vi "S4GUI_002.vi"(7 "Tab ObsEng":enum32{"Obs", "CCD modes", "Eng"}(tab)) -> ()   [LabVIEW 2018] (continued)
            n1927 = call-dynamic "Write sequencia_ant.vi"("error in (no error)"=w3775, "sequencia_ant"=w3776, "Opt_Selector in"=w3778) -> ("error out"=w3774:errorcluster, "Opt_Selector out"=w3777:refnum<class "Opt_Selector.lvclass">)  [unwired: 7 in]
            n1928 = local write "P8"(w3783) -> ()
            n1929 = local write "P9"(w3783) -> ()
            n1930 = local write "P10"(w3783) -> ()
            n1931 = local write "P11"(w3783) -> ()
            n1932 = local write "P12"(w3781) -> ()
            n1933 = local write "P13"(w3781) -> ()
            n1934 = local write "P14"(w3781) -> ()
            n1935 = local write "P15"(w3781) -> ()
          }
          frame 1 {
            w3787 = u16 255 ("sequencia")
            w3794 = FALSE ("P0")
            w3795 = TRUE ("P0")
            w3796 = FALSE ("P0")
            w3797 = TRUE ("P0")
            # "0000 0000 1111 1111 = 255"
            n1936 = local write "P0"(w3797) -> ()
            n1937 = local write "P1"(w3797) -> ()
            n1938 = local write "P2"(w3797) -> ()
            n1939 = local write "P3"(w3797) -> ()
            n1940 = local write "P4"(w3795) -> ()
            n1941 = local write "P5"(w3795) -> ()
            n1942 = local write "P6"(w3795) -> ()
            n1943 = local write "P7"(w3795) -> ()
            n1944 = call-dynamic "Write sequencia.vi"("error in (no error)"=w3792, "sequencia"=w3787, "Opt_Selector in"=w3793) -> ("error out"=w3789:errorcluster, "Opt_Selector out"=w3791:refnum<class "Opt_Selector.lvclass">)  [unwired: 7 in]
            n1945 = local write "P8"(w3796) -> ()
            n1946 = local write "P9"(w3796) -> ()
            n1947 = local write "P10"(w3796) -> ()
            n1948 = local write "P11"(w3796) -> ()
            n1949 = local write "P12"(w3794) -> ()
            n1950 = local write "P13"(w3794) -> ()
            n1951 = local write "P14"(w3794) -> ()
            n1952 = local write "P15"(w3794) -> ()
            n1953 = call-dynamic "Write sequencia_ant.vi"("error in (no error)"=w3789, "sequencia_ant"=w3787, "Opt_Selector in"=w3791) -> ("error out"=w3788:errorcluster, "Opt_Selector out"=w3790:refnum<class "Opt_Selector.lvclass">)  [unwired: 7 in]
          }
          frame 2 {
            w3800 = u16 15 ("sequencia")
            w3807 = FALSE ("P0")
            w3808 = FALSE ("P0")
            w3809 = FALSE ("P0")
            w3810 = TRUE ("P0")
            # "0000 0000 0000 1111 = 15"
            n1954 = local write "P0"(w3810) -> ()
            n1955 = local write "P1"(w3810) -> ()
            n1956 = local write "P2"(w3810) -> ()
            n1957 = local write "P3"(w3810) -> ()
            n1958 = local write "P4"(w3808) -> ()
            n1959 = local write "P5"(w3808) -> ()
            n1960 = local write "P6"(w3808) -> ()
            n1961 = local write "P7"(w3808) -> ()
            n1962 = call-dynamic "Write sequencia.vi"("error in (no error)"=w3805, "sequencia"=w3800, "Opt_Selector in"=w3806) -> ("error out"=w3802:errorcluster, "Opt_Selector out"=w3804:refnum<class "Opt_Selector.lvclass">)  [unwired: 7 in]
            n1963 = call-dynamic "Write sequencia_ant.vi"("error in (no error)"=w3802, "sequencia_ant"=w3800, "Opt_Selector in"=w3804) -> ("error out"=w3801:errorcluster, "Opt_Selector out"=w3803:refnum<class "Opt_Selector.lvclass">)  [unwired: 7 in]
            n1964 = local write "P8"(w3809) -> ()
            n1965 = local write "P9"(w3809) -> ()
            n1966 = local write "P10"(w3809) -> ()
            n1967 = local write "P11"(w3809) -> ()
            n1968 = local write "P12"(w3807) -> ()
            n1969 = local write "P13"(w3807) -> ()
            n1970 = local write "P14"(w3807) -> ()
            n1971 = local write "P15"(w3807) -> ()
          }
          frame 3 {
            w3814 = u16 3855 ("sequencia")
            w3820 = FALSE ("P0")
            w3821 = FALSE ("P0")
            w3822 = TRUE ("P0")
            w3823 = TRUE ("P0")
            # "0000 1111 0000 1111 = 3855"
            n1972 = local write "P0"(w3823) -> ()
            n1973 = local write "P1"(w3823) -> ()
            n1974 = local write "P2"(w3823) -> ()
            n1975 = local write "P3"(w3823) -> ()
            n1976 = local write "P4"(w3821) -> ()
            n1977 = local write "P5"(w3821) -> ()
            n1978 = local write "P6"(w3821) -> ()
            n1979 = local write "P7"(w3821) -> ()
            n1980 = call-dynamic "Write sequencia.vi"("error in (no error)"=w3818, "sequencia"=w3814, "Opt_Selector in"=w3819) -> ("error out"=w3816:errorcluster, "Opt_Selector out"=w3817:refnum<class "Opt_Selector.lvclass">)  [unwired: 7 in]
            n1981 = local write "P8"(w3822) -> ()
            n1982 = local write "P9"(w3822) -> ()
            n1983 = local write "P10"(w3822) -> ()
            n1984 = local write "P11"(w3822) -> ()
            n1985 = local write "P12"(w3820) -> ()
            n1986 = local write "P13"(w3820) -> ()
            n1987 = local write "P14"(w3820) -> ()
            n1988 = local write "P15"(w3820) -> ()
            n1989 = call-dynamic "Write sequencia_ant.vi"("error in (no error)"=w3816, "sequencia_ant"=w3814, "Opt_Selector in"=w3817) -> ("error out"=w3815:errorcluster, "Opt_Selector out"=w3813:refnum<class "Opt_Selector.lvclass">)  [unwired: 7 in]
          }
          frame 4 {
            w3826 = u16 0 ("sequencia")
            w3833 = FALSE ("P0")
            w3834 = FALSE ("P0")
            w3835 = FALSE ("P0")
            w3836 = FALSE ("P0")
            n1990 = local write "P0"(w3836) -> ()
            n1991 = local write "P1"(w3836) -> ()
            n1992 = local write "P2"(w3836) -> ()
            n1993 = local write "P3"(w3836) -> ()
            n1994 = local write "P4"(w3834) -> ()
            n1995 = local write "P5"(w3834) -> ()
            n1996 = local write "P6"(w3834) -> ()
            n1997 = local write "P7"(w3834) -> ()
            n1998 = call-dynamic "Write sequencia.vi"("error in (no error)"=w3831, "sequencia"=w3826, "Opt_Selector in"=w3832) -> ("error out"=w3828:errorcluster, "Opt_Selector out"=w3830:refnum<class "Opt_Selector.lvclass">)  [unwired: 7 in]
            n1999 = call-dynamic "Write sequencia_ant.vi"("error in (no error)"=w3828, "sequencia_ant"=w3826, "Opt_Selector in"=w3830) -> ("error out"=w3827:errorcluster, "Opt_Selector out"=w3829:refnum<class "Opt_Selector.lvclass">)  [unwired: 7 in]
            n2000 = local write "P8"(w3835) -> ()
            n2001 = local write "P9"(w3835) -> ()
            n2002 = local write "P10"(w3835) -> ()
            n2003 = local write "P11"(w3835) -> ()
            n2004 = local write "P12"(w3833) -> ()
            n2005 = local write "P13"(w3833) -> ()
            n2006 = local write "P14"(w3833) -> ()
            n2007 = local write "P15"(w3833) -> ()
          }
          frame 5 {
          }
        }
        n2008 = call "Write WPROT.vi"("error in (no error)"=w3733, "Opt_Selector.lvclass"=w3740, "Instrument in"=w3739) -> ("error out"=w3742:errorcluster, "Instrument out"=w3743:refnum<class "Instrument.lvclass">)  [unwired: 7 in]
        n2009 = property on="#Pol. Seq. Done" class="Slide (strict)"(error in=w3733, "Scale.Maximum"=w3734, "Scale.Minimum"=w3732) -> ()  [unwired: 1 in, 2 out]
        n2010 = call "Write Instrument.lvclass.vi"("error in (no error)"=w3742, "Instrument.lvclass"=w3743, "S4ACS_GUI in"=w3738) -> ("error out"=w3722:errorcluster, "S4ACS_GUI out"=w3723:refnum<class "S4GUI.lvclass">)  [unwired: 7 in]
        n2011 = call "Read Instrument.lvclass.vi"("error in (no error)"=w3722, "S4ACS_GUI in"=w3723) -> ("error out"=w3727:errorcluster, "Instrument.lvclass"=w3728:refnum<class "Instrument.lvclass">, "S4ACS_GUI out"=w3731:refnum<class "S4GUI.lvclass">)  [unwired: 7 in]
        n2012 = call "Read ASEL.vi"("error in (no error)"=w3727, "Instrument in"=w3728) -> ("error out"=w3717:errorcluster, "Opt_Selector.lvclass"=w3719:refnum<class "Opt_Selector.lvclass">, "Instrument out"=w3724:refnum<class "Instrument.lvclass">)  [unwired: 7 in]
        n2013 = call "Read name_pos.vi"("error in (no error)"=w3717, "Optics in"=w3719) -> ("error out"=w3716:errorcluster, "name_pos"=w3715:string, "Optics out"=w3718:refnum<class "Opt_Selector.lvclass">)  [unwired: 7 in]
        n2014 = call "Write ASEL.vi"("error in (no error)"=w3716, "Opt_Selector.lvclass"=w3718, "Instrument in"=w3724) -> ("error out"=w3725:errorcluster, "Instrument out"=w3729:refnum<class "Instrument.lvclass">)  [unwired: 7 in]
        n2015 = case shown="\"ON\"" w3715 {
          tunnel: w3725 -> [w3748 w3759]
          tunnel: [w3748 w3755] -> w3726
          tunnel: w3729 -> [w3747 w3760]
          tunnel: [w3747 w3756] -> w3730
          frame Default {
          }
          frame "ON" {
            n2016 = call "Read WPROT.vi"("error in (no error)"=w3759, "Instrument in"=w3760) -> ("error out"=w3751:errorcluster, "Opt_Selector.lvclass"=w3758:refnum<class "Opt_Selector.lvclass">, "Instrument out"=w3757:refnum<class "Instrument.lvclass">)  [unwired: 7 in]
            n2017 = call-dynamic "Read sequencia.vi"("error in (no error)"=w3751, "Opt_Selector in"=w3758) -> ("error out"=w3750:errorcluster, "sequencia"=w3754:u16, "Opt_Selector out"=w3753:refnum<class "Opt_Selector.lvclass">)  [unwired: 7 in]
            n2018 = case shown="0" w3754 {
              tunnel: w3753 -> [w3762 w3771]
              tunnel: [w3762 w3767] -> w3752
              tunnel: w3750 -> [w3761 w3770]
              tunnel: [w3761 w3765] -> w3749
              frame Default {
              }
              frame 0 {
                n2019 = call-dynamic "Write sequencia.vi"("error in (no error)"=w3770, "sequencia"=u16 1, "Opt_Selector in"=w3771) -> ("error out"=w3766:errorcluster, "Opt_Selector out"=w3768:refnum<class "Opt_Selector.lvclass">)  [unwired: 7 in]
                n2020 = local write "P0"(TRUE ("P0")) -> ()
                n2021 = call-dynamic "Write sequencia_ant.vi"("error in (no error)"=w3766, "sequencia_ant"=u16 1, "Opt_Selector in"=w3768) -> ("error out"=w3765:errorcluster, "Opt_Selector out"=w3767:refnum<class "Opt_Selector.lvclass">)  [unwired: 7 in]
              }
            }
            n2022 = call "Write WPROT.vi"("error in (no error)"=w3749, "Opt_Selector.lvclass"=w3752, "Instrument in"=w3757) -> ("error out"=w3755:errorcluster, "Instrument out"=w3756:refnum<class "Instrument.lvclass">)  [unwired: 7 in]
          }
        }
        n2023 = call "Write Instrument.lvclass.vi"("error in (no error)"=w3726, "Instrument.lvclass"=w3730, "S4ACS_GUI in"=w3731) -> ("error out"=w3721:errorcluster, "S4ACS_GUI out"=w3720:refnum<class "S4GUI.lvclass">)  [unwired: 7 in]
      }
      event "P0", "P1", "P2", "P3", "P4", "P5", "P6", "P7", "P8", "P9", "P10", "P11", "P12", "P13", "P14", "P15": Value Change {
        w3894 = u16 5 items=["All 16 positions", "First 8 positions", "First 4 positions", "0-3 + 8-11", "Clear", "Customized"] ("Select Positions")
        # "Garantir que, quando em POLARIMETRIA, pelo menos WP1 esteja selecionado."
        # "Salva tambem em \nSequencia_ant para\no caso de repeticao."
        n2024 = event-data() -> ()  [unwired: 1 in, 6 out]
        n2025 = call "Read Instrument.lvclass.vi"("error in (no error)"=w3876, "S4ACS_GUI in"=w3877) -> ("error out"=w3871:errorcluster, "Instrument.lvclass"=w3874:refnum<class "Instrument.lvclass">, "S4ACS_GUI out"=w3875:refnum<class "S4GUI.lvclass">)  [unwired: 7 in]
        n2026 = Build Array("P0", "P1", "P2", "P3", "P4", "P5", "P6", "P7", "P8", "P9", "P10", "P11", "P12", "P13", "P14", "P15") -> (w3862:bool[])
        n2027 = call "Read WPROT.vi"("error in (no error)"=w3871, "Instrument in"=w3874) -> ("error out"=w3870:errorcluster, "Opt_Selector.lvclass"=w3872:refnum<class "Opt_Selector.lvclass">, "Instrument out"=w3873:refnum<class "Instrument.lvclass">)  [unwired: 7 in]
        n2028 = local write "Select Positions"(w3894) -> ()
        n2029 = Boolean Array To Number(Boolean array=w3862) -> (number=w3878:u32)
        n2030 = To Unsigned Word Integer(number=w3878) -> (unsigned 16bit integer=w3863:u16)
        n2031 = call-dynamic "Write sequencia.vi"("error in (no error)"=w3870, "sequencia"=w3863, "Opt_Selector in"=w3872) -> ("error out"=w3865:errorcluster, "Opt_Selector out"=w3867:refnum<class "Opt_Selector.lvclass">)  [unwired: 7 in]
        n2032 = call-dynamic "Write sequencia_ant.vi"("error in (no error)"=w3865, "sequencia_ant"=w3863, "Opt_Selector in"=w3867) -> ("error out"=w3864:errorcluster, "Opt_Selector out"=w3866:refnum<class "Opt_Selector.lvclass">)  [unwired: 7 in]
        n2033 = for {
          tunnel: w3862 -> [w3923] mode=indexing
          shift-right: [w3922] -> w3860
          shift-left: 0 -> [w3920]
          # "calcula qtd de 1s"
          n2034 = Increment(x=w3920) -> (x+1=w3921:i32)
          n2035 = Select(t=w3921, s=w3923, f=w3920) -> (s? t:f=w3922:i32)
        }
        n2036 = call "Write WPROT.vi"("error in (no error)"=w3864, "Opt_Selector.lvclass"=w3866, "Instrument in"=w3873) -> ("error out"=w3869:errorcluster, "Instrument out"=w3868:refnum<class "Instrument.lvclass">)  [unwired: 7 in]
        n2037 = call "Write Instrument.lvclass.vi"("error in (no error)"=w3869, "Instrument.lvclass"=w3868, "S4ACS_GUI in"=w3875) -> ("error out"=w3843:errorcluster, "S4ACS_GUI out"=w3844:refnum<class "S4GUI.lvclass">)  [unwired: 7 in]
        n2038 = property on="#Pol. Seq. Done" class="Slide (strict)"("Scale.Maximum"=w3860, "Scale.Minimum"=0.0 ("Scale.Range:Minimum")) -> ()  [unwired: 2 in, 2 out]
        n2039 = call "Read Instrument.lvclass.vi"("error in (no error)"=w3843, "S4ACS_GUI in"=w3844) -> ("error out"=w3849:errorcluster, "Instrument.lvclass"=w3848:refnum<class "Instrument.lvclass">, "S4ACS_GUI out"=w3845:refnum<class "S4GUI.lvclass">)  [unwired: 7 in]
        n2040 = call "Read ASEL.vi"("error in (no error)"=w3849, "Instrument in"=w3848) -> ("error out"=w3855:errorcluster, "Opt_Selector.lvclass"=w3853:refnum<class "Opt_Selector.lvclass">, "Instrument out"=w3852:refnum<class "Instrument.lvclass">)  [unwired: 7 in]
        n2041 = call "Read name_pos.vi"("error in (no error)"=w3855, "Optics in"=w3853) -> ("error out"=w3856:errorcluster, "name_pos"=w3857:string, "Optics out"=w3854:refnum<class "Opt_Selector.lvclass">)  [unwired: 7 in]
        n2042 = call "Write ASEL.vi"("error in (no error)"=w3856, "Opt_Selector.lvclass"=w3854, "Instrument in"=w3852) -> ("error out"=w3851:errorcluster, "Instrument out"=w3847:refnum<class "Instrument.lvclass">)  [unwired: 7 in]
        n2043 = case shown="\"ON\"" w3857 {
          tunnel: w3851 -> [w3896 w3907]
          tunnel: [w3896 w3903] -> w3850
          tunnel: w3847 -> [w3895 w3908]
          tunnel: [w3895 w3904] -> w3846
          frame Default {
          }
          frame "ON" {
            n2044 = call "Read WPROT.vi"("error in (no error)"=w3907, "Instrument in"=w3908) -> ("error out"=w3899:errorcluster, "Opt_Selector.lvclass"=w3906:refnum<class "Opt_Selector.lvclass">, "Instrument out"=w3905:refnum<class "Instrument.lvclass">)  [unwired: 7 in]
            n2045 = call-dynamic "Read sequencia.vi"("error in (no error)"=w3899, "Opt_Selector in"=w3906) -> ("error out"=w3898:errorcluster, "sequencia"=w3902:u16, "Opt_Selector out"=w3901:refnum<class "Opt_Selector.lvclass">)  [unwired: 7 in]
            n2046 = case shown="0" w3902 {
              tunnel: w3901 -> [w3910 w3919]
              tunnel: [w3910 w3915] -> w3900
              tunnel: w3898 -> [w3909 w3918]
              tunnel: [w3909 w3913] -> w3897
              frame Default {
              }
              frame 0 {
                n2047 = call-dynamic "Write sequencia.vi"("error in (no error)"=w3918, "sequencia"=u16 1, "Opt_Selector in"=w3919) -> ("error out"=w3914:errorcluster, "Opt_Selector out"=w3916:refnum<class "Opt_Selector.lvclass">)  [unwired: 7 in]
                n2048 = local write "P0"(TRUE ("P0")) -> ()
                n2049 = call-dynamic "Write sequencia_ant.vi"("error in (no error)"=w3914, "sequencia_ant"=u16 1, "Opt_Selector in"=w3916) -> ("error out"=w3913:errorcluster, "Opt_Selector out"=w3915:refnum<class "Opt_Selector.lvclass">)  [unwired: 7 in]
              }
            }
            n2050 = call "Write WPROT.vi"("error in (no error)"=w3897, "Opt_Selector.lvclass"=w3900, "Instrument in"=w3905) -> ("error out"=w3903:errorcluster, "Instrument out"=w3904:refnum<class "Instrument.lvclass">)  [unwired: 7 in]
          }
        }
        n2051 = call "Write Instrument.lvclass.vi"("error in (no error)"=w3850, "Instrument.lvclass"=w3846, "S4ACS_GUI in"=w3845) -> ("error out"=w3841:errorcluster, "S4ACS_GUI out"=w3842:refnum<class "S4GUI.lvclass">)  [unwired: 7 in]
      }
      event "SSM": Value Change {
        # "F: fotom.\nT: polar."
        n2052 = event-data() -> ("NewVal"=w3931:u16)  [unwired: 1 in, 5 out]
        n2053 = call-dynamic "Read mode EXPOSE.vi"("error in (no error)"=w3937, "S4GUI in"=w3938) -> ("error out"=w3936:errorcluster, "mode EXPOSE"=w3932:bool, "S4GUI out"=w3933:refnum<class "S4GUI.lvclass">)  [unwired: 7 in]
        n2054 = call "Read Instrument.lvclass.vi"("error in (no error)"=w3936, "S4ACS_GUI in"=w3933) -> ("error out"=w3935:errorcluster, "Instrument.lvclass"=w3941:refnum<class "Instrument.lvclass">, "S4ACS_GUI out"=w3940:refnum<class "S4GUI.lvclass">)  [unwired: 7 in]
        n2055 = call-dynamic "Read mode.vi"("error in (no error)"=w3935, "Instrument in"=w3941) -> ("error out"=w3934:errorcluster, "mode"=w3939:bool)  [unwired: 7 in, 1 out]
        n2056 = case shown="1" w3931 {
          tunnel: [TRUE FALSE] -> w3944
          tunnel: w3934 -> [w3950 w4177]
          tunnel: w3940 -> [w3952 w4176]
          tunnel: [w3954 w4168] -> w3943
          tunnel: [w3946 w4167] -> w3942
          tunnel: w3939 -> [_ w4157]
          tunnel: w3932 -> [_ w4155]
          tunnel: ["SYNCHRONOUS" "ASYNCHRONOUS"] -> w3924
          frame 1 {
            # "Sync mode: Os canais sao configurados para Trigger externo, desde que o SyncBox esteja conectado."
            # "Sync by Cycle"
            n2057 = call-dynamic "Read Sync Box.lvclass.vi"("error in (no error)"=w3950, "SPARC4_AC in"=w3952) -> ("error out"=w3949:errorcluster, "Sync Box.lvclass"=w3953:refnum<class "Sync Box.lvclass">, "SPARC4_AC out"=w3951:refnum<class "S4GUI.lvclass">)  [unwired: 7 in]
            n2058 = call "Read connection.vi"("error in (no error)"=w3949, "Server in"=w3953) -> ("error out"=w3948:errorcluster, "connection"=w3947:bool)  [unwired: 7 in, 1 out]
            n2059 = case shown="False" w3947 {
              tunnel: [w3957 w3974] -> w3954
              tunnel: w3951 -> [w3957 w3964]
              tunnel: w3948 -> [w3956 w3963]
              tunnel: [w3956 w3958] -> w3946
              frame False {
              }
              frame True {
                n2060 = call-dynamic "Read AcquisitionC.vi"("error in (no error)"=w3963, "S4ACS_GUI in"=w3964) -> ("error out"=w3981:errorcluster, "Acquisition.lvclass"=w3980:refnum<class "Acquisition.lvclass">)  [unwired: 7 in, 1 out]
                n2061 = call-dynamic "Read AcquisitionA.vi"("error in (no error)"=w3963, "S4ACS_GUI in"=w3964) -> ("error out"=w3984:errorcluster, "Acquisition.lvclass"=w3985:refnum<class "Acquisition.lvclass">, "S4ACS_GUI out"=w3973:refnum<class "S4GUI.lvclass">)  [unwired: 7 in]
                n2062 = call "Read AcquisitionB.vi"("error in (no error)"=w3963, "S4ACS_GUI in"=w3964) -> ("error out"=w3982:errorcluster, "Acquisition.lvclass"=w3983:refnum<class "Acquisition.lvclass">)  [unwired: 7 in, 1 out]
                n2063 = call-dynamic "Read AcquisitionD.vi"("error in (no error)"=w3963, "S4ACS_GUI in"=w3964) -> ("error out"=w3978:errorcluster, "Acquisition.lvclass"=w3979:refnum<class "Acquisition.lvclass">)  [unwired: 7 in, 1 out]
                n2064 = call-dynamic "Read enabled.vi"("error in (no error)"=w3978, "Server in"=w3979) -> ("error out"=w3987:errorcluster, "enabled"=w3986:bool, "Server out"=w3988:refnum<class "Acquisition.lvclass">)  [unwired: 7 in]
                n2065 = call-dynamic "Read enabled.vi"("error in (no error)"=w3981, "Server in"=w3980) -> ("error out"=w3990:errorcluster, "enabled"=w3989:bool, "Server out"=w3991:refnum<class "Acquisition.lvclass">)  [unwired: 7 in]
                n2066 = call-dynamic "Read enabled.vi"("error in (no error)"=w3982, "Server in"=w3983) -> ("error out"=w3993:errorcluster, "enabled"=w3992:bool, "Server out"=w3994:refnum<class "Acquisition.lvclass">)  [unwired: 7 in]
                n2067 = call-dynamic "Read enabled.vi"("error in (no error)"=w3984, "Server in"=w3985) -> ("error out"=w3996:errorcluster, "enabled"=w3995:bool, "Server out"=w3997:refnum<class "Acquisition.lvclass">)  [unwired: 7 in]
                n2068 = case shown="True" w3992 {
                  tunnel: w3994 -> [w4077 w4081]
                  tunnel: w3993 -> [w4076 w4080]
                  tunnel: [w4077 w4079] -> w3970
                  tunnel: [w4076 w4078] -> w3969
                  frame False {
                  }
                  frame True {
                    # "Ext Start"
                    # "nome do arquivo .cfg"
                    # "seção no arquivo .cfg"
                    n2069 = call-dynamic "Read Channel.vi"("error in (no error)"=w4080, "Acquisition in"=w4081) -> ("error out"=w4085:errorcluster, "Channel.lvclass"=w4084:refnum<class "Channel.lvclass">, "Acquisition out"=w4083:refnum<class "Acquisition.lvclass">)  [unwired: 7 in]
                    n2070 = call-dynamic "Read Interface.vi"("error in (no error)"=w4085, "Channel in"=w4084) -> ("error out"=w4093:errorcluster, "Interface.lvclass"=w4094:refnum<class "Interface.lvclass">, "Channel out"=w4082:refnum<class "Channel.lvclass">)  [unwired: 7 in]
                    n2071 = call-dynamic "Get CCD_Config.vi"("error in (no error)"=w4093, "Interface in"=w4094) -> ("error out"=w4090:errorcluster, "output cluster"=w4089:T31, "Interface out"=w4095:refnum<class "Interface.lvclass">)  [unwired: 7 in]
                    n2072 = Bundle By Name(cluster=w4089, "TRIGGER_MODE"=u8 6 ("SHUTTER_MODE")) -> (w4091:T31)
                    n2073 = call-dynamic "Set CCD_Config.vi"("error in (no error)"=w4090, "input cluster"=w4091, "Interface in"=w4095) -> ("error out"=w4088:errorcluster, "Interface out"=w4096:refnum<class "Interface.lvclass">)  [unwired: 7 in]
                    n2074 = Flatten To String(anything=w4091, error in (no error)=w4088) -> (data string=w4086:string, error out=w4087:errorcluster)  [unwired: 2 in, 1 out]
                    n2075 = call "Write flatted cluster.vi"("error in (no error)"=w4087, "flatted cluster"=w4086, "Interface in"=w4096) -> ("error out"=w4098:errorcluster, "Interface out"=w4097:refnum<class "Interface.lvclass">)  [unwired: 7 in]
                    n2076 = call-dynamic "Write Interface.vi"("error in (no error)"=w4098, "Interface.lvclass"=w4097, "Channel in"=w4082) -> ("error out"=w4104:errorcluster, "Channel out"=w4105:refnum<class "Channel.lvclass">)  [unwired: 7 in]
                    n2077 = call "Write section_name.vi"("error in (no error)"=w4104, "section_name"="CCD_ACS2", "Channel in"=w4105) -> ("error out"=w4102:errorcluster, "Channel out"=w4108:refnum<class "Channel.lvclass">)  [unwired: 7 in]
                    n2078 = call-dynamic "save config.vi"("error in (no error)"=w4102, "file config"="lastsaved.cfg", "Channel in"=w4108) -> ("error out"=w4103:errorcluster, "Channel out"=w4109:refnum<class "Channel.lvclass">)  [unwired: 7 in]
                    n2079 = call-dynamic "Read State Machine.vi"("error in (no error)"=w4103, "Device in"=w4109) -> ("error out"=w4099:errorcluster, "State Machine.lvclass"=w4111:refnum<class "State Machine.lvclass">, "Device out"=w4110:refnum<class "Channel.lvclass">)  [unwired: 7 in]
                    n2080 = call-dynamic "Write State.vi"("error in (no error)"=w4099, "State"=60, "State Machine in"=w4111) -> ("error out"=w4100:errorcluster, "State Machine out"=w4112:refnum<class "State Machine.lvclass">)  [unwired: 7 in]
                    n2081 = call-dynamic "Write State Machine.vi"("error in (no error)"=w4100, "State Machine.lvclass"=w4112, "Device in"=w4110) -> ("error out"=w4114:errorcluster, "Device out"=w4113:refnum<class "Channel.lvclass">)  [unwired: 7 in]
                    n2082 = call-dynamic "Write Channel.vi"("error in (no error)"=w4114, "Channel.lvclass"=w4113, "Acquisition in"=w4083) -> ("error out"=w4078:errorcluster, "Acquisition out"=w4079:refnum<class "Acquisition.lvclass">)  [unwired: 7 in]
                  }
                }
                n2083 = case shown="True" w3995 {
                  tunnel: [w4115 w4149] -> w3971
                  tunnel: [w4116 w4148] -> w3972
                  tunnel: w3997 -> [w4116 w4118]
                  tunnel: w3996 -> [w4115 w4117]
                  frame False {
                  }
                  frame True {
                    # "nome do arquivo .cfg"
                    # "seção no arquivo .cfg"
                    # "Ext Start"
                    n2084 = call-dynamic "Read Channel.vi"("error in (no error)"=w4117, "Acquisition in"=w4118) -> ("error out"=w4150:errorcluster, "Channel.lvclass"=w4151:refnum<class "Channel.lvclass">, "Acquisition out"=w4152:refnum<class "Acquisition.lvclass">)  [unwired: 7 in]
                    n2085 = call-dynamic "Read Interface.vi"("error in (no error)"=w4150, "Channel in"=w4151) -> ("error out"=w4140:errorcluster, "Interface.lvclass"=w4139:refnum<class "Interface.lvclass">, "Channel out"=w4153:refnum<class "Channel.lvclass">)  [unwired: 7 in]
                    n2086 = call-dynamic "Get CCD_Config.vi"("error in (no error)"=w4140, "Interface in"=w4139) -> ("error out"=w4143:errorcluster, "output cluster"=w4144:T31, "Interface out"=w4138:refnum<class "Interface.lvclass">)  [unwired: 7 in]
                    n2087 = Bundle By Name(cluster=w4144, "TRIGGER_MODE"=u8 6 ("SHUTTER_MODE")) -> (w4142:T31)
                    n2088 = call-dynamic "Set CCD_Config.vi"("error in (no error)"=w4143, "input cluster"=w4142, "Interface in"=w4138) -> ("error out"=w4145:errorcluster, "Interface out"=w4137:refnum<class "Interface.lvclass">)  [unwired: 7 in]
                    n2089 = Flatten To String(anything=w4142, error in (no error)=w4145) -> (data string=w4147:string, error out=w4146:errorcluster)  [unwired: 2 in, 1 out]
                    n2090 = call "Write flatted cluster.vi"("error in (no error)"=w4146, "flatted cluster"=w4147, "Interface in"=w4137) -> ("error out"=w4135:errorcluster, "Interface out"=w4136:refnum<class "Interface.lvclass">)  [unwired: 7 in]
                    n2091 = call-dynamic "Write Interface.vi"("error in (no error)"=w4135, "Interface.lvclass"=w4136, "Channel in"=w4153) -> ("error out"=w4130:errorcluster, "Channel out"=w4129:refnum<class "Channel.lvclass">)  [unwired: 7 in]
                    n2092 = call "Write section_name.vi"("error in (no error)"=w4130, "section_name"="CCD_ACS1", "Channel in"=w4129) -> ("error out"=w4131:errorcluster, "Channel out"=w4126:refnum<class "Channel.lvclass">)  [unwired: 7 in]
                    n2093 = call-dynamic "save config.vi"("error in (no error)"=w4131, "file config"="lastsaved.cfg", "Channel in"=w4126) -> ("error out"=w4119:errorcluster, "Channel out"=w4120:refnum<class "Channel.lvclass">)  [unwired: 7 in]
                    n2094 = call-dynamic "Read State Machine.vi"("error in (no error)"=w4119, "Device in"=w4120) -> ("error out"=w4134:errorcluster, "State Machine.lvclass"=w4124:refnum<class "State Machine.lvclass">, "Device out"=w4125:refnum<class "Channel.lvclass">)  [unwired: 7 in]
                    n2095 = call-dynamic "Write State.vi"("error in (no error)"=w4134, "State"=60, "State Machine in"=w4124) -> ("error out"=w4133:errorcluster, "State Machine out"=w4123:refnum<class "State Machine.lvclass">)  [unwired: 7 in]
                    n2096 = call-dynamic "Write State Machine.vi"("error in (no error)"=w4133, "State Machine.lvclass"=w4123, "Device in"=w4125) -> ("error out"=w4121:errorcluster, "Device out"=w4122:refnum<class "Channel.lvclass">)  [unwired: 7 in]
                    n2097 = call-dynamic "Write Channel.vi"("error in (no error)"=w4121, "Channel.lvclass"=w4122, "Acquisition in"=w4152) -> ("error out"=w4149:errorcluster, "Acquisition out"=w4148:refnum<class "Acquisition.lvclass">)  [unwired: 7 in]
                  }
                }
                n2098 = case shown="True" w3989 {
                  tunnel: w3991 -> [w4038 w4042]
                  tunnel: w3990 -> [w4037 w4041]
                  tunnel: [w4038 w4040] -> w3968
                  tunnel: [w4037 w4039] -> w3967
                  frame False {
                  }
                  frame True {
                    # "Ext Start"
                    # "nome do arquivo .cfg"
                    # "seção no arquivo .cfg"
                    n2099 = call-dynamic "Read Channel.vi"("error in (no error)"=w4041, "Acquisition in"=w4042) -> ("error out"=w4046:errorcluster, "Channel.lvclass"=w4045:refnum<class "Channel.lvclass">, "Acquisition out"=w4044:refnum<class "Acquisition.lvclass">)  [unwired: 7 in]
                    n2100 = call-dynamic "Read Interface.vi"("error in (no error)"=w4046, "Channel in"=w4045) -> ("error out"=w4054:errorcluster, "Interface.lvclass"=w4055:refnum<class "Interface.lvclass">, "Channel out"=w4043:refnum<class "Channel.lvclass">)  [unwired: 7 in]
                    n2101 = call-dynamic "Get CCD_Config.vi"("error in (no error)"=w4054, "Interface in"=w4055) -> ("error out"=w4051:errorcluster, "output cluster"=w4050:T31, "Interface out"=w4056:refnum<class "Interface.lvclass">)  [unwired: 7 in]
                    n2102 = Bundle By Name(cluster=w4050, "TRIGGER_MODE"=u8 6 ("SHUTTER_MODE")) -> (w4052:T31)
                    n2103 = call-dynamic "Set CCD_Config.vi"("error in (no error)"=w4051, "input cluster"=w4052, "Interface in"=w4056) -> ("error out"=w4049:errorcluster, "Interface out"=w4057:refnum<class "Interface.lvclass">)  [unwired: 7 in]
                    n2104 = Flatten To String(anything=w4052, error in (no error)=w4049) -> (data string=w4047:string, error out=w4048:errorcluster)  [unwired: 2 in, 1 out]
                    n2105 = call "Write flatted cluster.vi"("error in (no error)"=w4048, "flatted cluster"=w4047, "Interface in"=w4057) -> ("error out"=w4059:errorcluster, "Interface out"=w4058:refnum<class "Interface.lvclass">)  [unwired: 7 in]
                    n2106 = call-dynamic "Write Interface.vi"("error in (no error)"=w4059, "Interface.lvclass"=w4058, "Channel in"=w4043) -> ("error out"=w4065:errorcluster, "Channel out"=w4066:refnum<class "Channel.lvclass">)  [unwired: 7 in]
                    n2107 = call "Write section_name.vi"("error in (no error)"=w4065, "section_name"="CCD_ACS3", "Channel in"=w4066) -> ("error out"=w4063:errorcluster, "Channel out"=w4069:refnum<class "Channel.lvclass">)  [unwired: 7 in]
                    n2108 = call-dynamic "save config.vi"("error in (no error)"=w4063, "file config"="lastsaved.cfg", "Channel in"=w4069) -> ("error out"=w4064:errorcluster, "Channel out"=w4070:refnum<class "Channel.lvclass">)  [unwired: 7 in]
                    n2109 = call-dynamic "Read State Machine.vi"("error in (no error)"=w4064, "Device in"=w4070) -> ("error out"=w4060:errorcluster, "State Machine.lvclass"=w4072:refnum<class "State Machine.lvclass">, "Device out"=w4071:refnum<class "Channel.lvclass">)  [unwired: 7 in]
                    n2110 = call-dynamic "Write State.vi"("error in (no error)"=w4060, "State"=60, "State Machine in"=w4072) -> ("error out"=w4061:errorcluster, "State Machine out"=w4073:refnum<class "State Machine.lvclass">)  [unwired: 7 in]
                    n2111 = call-dynamic "Write State Machine.vi"("error in (no error)"=w4061, "State Machine.lvclass"=w4073, "Device in"=w4071) -> ("error out"=w4075:errorcluster, "Device out"=w4074:refnum<class "Channel.lvclass">)  [unwired: 7 in]
                    n2112 = call-dynamic "Write Channel.vi"("error in (no error)"=w4075, "Channel.lvclass"=w4074, "Acquisition in"=w4044) -> ("error out"=w4039:errorcluster, "Acquisition out"=w4040:refnum<class "Acquisition.lvclass">)  [unwired: 7 in]
                  }
                }
                n2113 = case shown="True" w3986 {
                  tunnel: w3988 -> [w3999 w4003]
                  tunnel: w3987 -> [w3998 w4002]
                  tunnel: [w3999 w4001] -> w3966
                  tunnel: [w3998 w4000] -> w3965
                  frame False {
                  }
                  frame True {
                    # "Ext Start"
                    # "nome do arquivo .cfg"
                    # "seção no arquivo .cfg"
                    n2114 = call-dynamic "Read Channel.vi"("error in (no error)"=w4002, "Acquisition in"=w4003) -> ("error out"=w4033:errorcluster, "Channel.lvclass"=w4034:refnum<class "Channel.lvclass">, "Acquisition out"=w4035:refnum<class "Acquisition.lvclass">)  [unwired: 7 in]
                    n2115 = call-dynamic "Read Interface.vi"("error in (no error)"=w4033, "Channel in"=w4034) -> ("error out"=w4025:errorcluster, "Interface.lvclass"=w4024:refnum<class "Interface.lvclass">, "Channel out"=w4036:refnum<class "Channel.lvclass">)  [unwired: 7 in]
                    n2116 = call-dynamic "Get CCD_Config.vi"("error in (no error)"=w4025, "Interface in"=w4024) -> ("error out"=w4028:errorcluster, "output cluster"=w4029:T31, "Interface out"=w4023:refnum<class "Interface.lvclass">)  [unwired: 7 in]
                    n2117 = Bundle By Name(cluster=w4029, "TRIGGER_MODE"=u8 6 ("SHUTTER_MODE")) -> (w4027:T31)
                    n2118 = call-dynamic "Set CCD_Config.vi"("error in (no error)"=w4028, "input cluster"=w4027, "Interface in"=w4023) -> ("error out"=w4030:errorcluster, "Interface out"=w4022:refnum<class "Interface.lvclass">)  [unwired: 7 in]
                    n2119 = Flatten To String(anything=w4027, error in (no error)=w4030) -> (data string=w4032:string, error out=w4031:errorcluster)  [unwired: 2 in, 1 out]
                    n2120 = call "Write flatted cluster.vi"("error in (no error)"=w4031, "flatted cluster"=w4032, "Interface in"=w4022) -> ("error out"=w4020:errorcluster, "Interface out"=w4021:refnum<class "Interface.lvclass">)  [unwired: 7 in]
                    n2121 = call-dynamic "Write Interface.vi"("error in (no error)"=w4020, "Interface.lvclass"=w4021, "Channel in"=w4036) -> ("error out"=w4014:errorcluster, "Channel out"=w4013:refnum<class "Channel.lvclass">)  [unwired: 7 in]
                    n2122 = call "Write section_name.vi"("error in (no error)"=w4014, "section_name"="CCD_ACS4", "Channel in"=w4013) -> ("error out"=w4016:errorcluster, "Channel out"=w4010:refnum<class "Channel.lvclass">)  [unwired: 7 in]
                    n2123 = call-dynamic "save config.vi"("error in (no error)"=w4016, "file config"="lastsaved.cfg", "Channel in"=w4010) -> ("error out"=w4015:errorcluster, "Channel out"=w4009:refnum<class "Channel.lvclass">)  [unwired: 7 in]
                    n2124 = call-dynamic "Read State Machine.vi"("error in (no error)"=w4015, "Device in"=w4009) -> ("error out"=w4019:errorcluster, "State Machine.lvclass"=w4007:refnum<class "State Machine.lvclass">, "Device out"=w4008:refnum<class "Channel.lvclass">)  [unwired: 7 in]
                    n2125 = call-dynamic "Write State.vi"("error in (no error)"=w4019, "State"=60, "State Machine in"=w4007) -> ("error out"=w4018:errorcluster, "State Machine out"=w4006:refnum<class "State Machine.lvclass">)  [unwired: 7 in]
                    n2126 = call-dynamic "Write State Machine.vi"("error in (no error)"=w4018, "State Machine.lvclass"=w4006, "Device in"=w4008) -> ("error out"=w4004:errorcluster, "Device out"=w4005:refnum<class "Channel.lvclass">)  [unwired: 7 in]
                    n2127 = call-dynamic "Write Channel.vi"("error in (no error)"=w4004, "Channel.lvclass"=w4005, "Acquisition in"=w4035) -> ("error out"=w4000:errorcluster, "Acquisition out"=w4001:refnum<class "Acquisition.lvclass">)  [unwired: 7 in]
                  }
                }
                n2128 = call-dynamic "Write AcquisitionA.vi"("error in (no error)"=w3971, "Acquisition.lvclass"=w3972, "S4ACS_GUI in"=w3973) -> ("error out"=w3962:errorcluster, "S4ACS_GUI out"=w3977:refnum<class "S4GUI.lvclass">)  [unwired: 7 in]
                n2129 = call "Write AcquisitionB.vi"("error in (no error)"=w3969, "Acquisition.lvclass"=w3970, "S4ACS_GUI in"=w3977) -> ("error out"=w3961:errorcluster, "S4ACS_GUI out"=w3976:refnum<class "S4GUI.lvclass">)  [unwired: 7 in]
                n2130 = call-dynamic "Write AcquisitionC.vi"("error in (no error)"=w3967, "Acquisition.lvclass"=w3968, "S4ACS_GUI in"=w3976) -> ("error out"=w3960:errorcluster, "S4ACS_GUI out"=w3975:refnum<class "S4GUI.lvclass">)  [unwired: 7 in]
                n2131 = call-dynamic "Write AcquisitionD.vi"("error in (no error)"=w3965, "Acquisition.lvclass"=w3966, "S4ACS_GUI in"=w3975) -> ("error out"=w3959:errorcluster, "S4ACS_GUI out"=w3974:refnum<class "S4GUI.lvclass">)  [unwired: 7 in]
                n2132 = Merge Errors(w3962, w3961, w3960, w3959) -> (w3958:errorcluster)
              }
            }
          }
          frame 0, Default {
            # "Async mode: Os canais são configurados com Trigger Interno para Fotometria ou Trigger Externo para Polarimetria (independentemente do status do SyncBox)"
            # "Aynchronous:"
            n2133 = call-dynamic "Read AcquisitionC.vi"("error in (no error)"=w4177, "S4ACS_GUI in"=w4176) -> ("error out"=w4181:errorcluster, "Acquisition.lvclass"=w4180:refnum<class "Acquisition.lvclass">)  [unwired: 7 in, 1 out]
            n2134 = call "Read AcquisitionB.vi"("error in (no error)"=w4177, "S4ACS_GUI in"=w4176) -> ("error out"=w4182:errorcluster, "Acquisition.lvclass"=w4183:refnum<class "Acquisition.lvclass">)  [unwired: 7 in, 1 out]
            n2135 = call-dynamic "Read AcquisitionA.vi"("error in (no error)"=w4177, "S4ACS_GUI in"=w4176) -> ("error out"=w4184:errorcluster, "Acquisition.lvclass"=w4185:refnum<class "Acquisition.lvclass">, "S4ACS_GUI out"=w4166:refnum<class "S4GUI.lvclass">)  [unwired: 7 in]
            n2136 = case shown="False" w4157 {
              tunnel: [u8 0 ("SHUTTER_MODE") w4200] -> w4156
              tunnel: w4155 -> [_ w4203]
              frame False {
                # "Fotom."
                # "Internal"
              }
              frame True {
                # "exp mode?"
                # "Internal"
                # "Polar."
                # "Ext. Start"
                n2137 = Select(t=u8 0, s=w4203, f=u8 6 ("SHUTTER_MODE")) -> (s? t:f=w4200:u8)
              }
            }
            n2138 = call-dynamic "Read AcquisitionD.vi"("error in (no error)"=w4177, "S4ACS_GUI in"=w4176) -> ("error out"=w4178:errorcluster, "Acquisition.lvclass"=w4179:refnum<class "Acquisition.lvclass">)  [unwired: 7 in, 1 out]
            n2139 = call-dynamic "Read enabled.vi"("error in (no error)"=w4181, "Server in"=w4180) -> ("error out"=w4190:errorcluster, "enabled"=w4189:bool, "Server out"=w4191:refnum<class "Acquisition.lvclass">)  [unwired: 7 in]
            n2140 = call-dynamic "Read enabled.vi"("error in (no error)"=w4182, "Server in"=w4183) -> ("error out"=w4193:errorcluster, "enabled"=w4192:bool, "Server out"=w4194:refnum<class "Acquisition.lvclass">)  [unwired: 7 in]
            n2141 = call-dynamic "Read enabled.vi"("error in (no error)"=w4178, "Server in"=w4179) -> ("error out"=w4187:errorcluster, "enabled"=w4186:bool, "Server out"=w4188:refnum<class "Acquisition.lvclass">)  [unwired: 7 in]
            n2142 = call-dynamic "Read enabled.vi"("error in (no error)"=w4184, "Server in"=w4185) -> ("error out"=w4196:errorcluster, "enabled"=w4195:bool, "Server out"=w4197:refnum<class "Acquisition.lvclass">)  [unwired: 7 in]
            n2143 = case shown="True" w4189 {
              tunnel: w4191 -> [w4244 w4249]
              tunnel: w4190 -> [w4243 w4248]
              tunnel: [w4244 w4247] -> w4161
              tunnel: [w4243 w4246] -> w4160
              tunnel: w4156 -> [_ w4245]
              frame False {
              }
              frame True {
                # "nome do arquivo .cfg"
                # "seção no arquivo .cfg"
                n2144 = call-dynamic "Read Channel.vi"("error in (no error)"=w4248, "Acquisition in"=w4249) -> ("error out"=w4253:errorcluster, "Channel.lvclass"=w4252:refnum<class "Channel.lvclass">, "Acquisition out"=w4251:refnum<class "Acquisition.lvclass">)  [unwired: 7 in]
                n2145 = call-dynamic "Read Interface.vi"("error in (no error)"=w4253, "Channel in"=w4252) -> ("error out"=w4260:errorcluster, "Interface.lvclass"=w4261:refnum<class "Interface.lvclass">, "Channel out"=w4250:refnum<class "Channel.lvclass">)  [unwired: 7 in]
                n2146 = call-dynamic "Get CCD_Config.vi"("error in (no error)"=w4260, "Interface in"=w4261) -> ("error out"=w4258:errorcluster, "output cluster"=w4257:T31, "Interface out"=w4262:refnum<class "Interface.lvclass">)  [unwired: 7 in]
                n2147 = Bundle By Name(cluster=w4257, "TRIGGER_MODE"=w4245) -> (w4259:T31)
                n2148 = call-dynamic "Set CCD_Config.vi"("error in (no error)"=w4258, "input cluster"=w4259, "Interface in"=w4262) -> ("error out"=w4256:errorcluster, "Interface out"=w4263:refnum<class "Interface.lvclass">)  [unwired: 7 in]
                n2149 = Flatten To String(anything=w4259, error in (no error)=w4256) -> (data string=w4254:string, error out=w4255:errorcluster)  [unwired: 2 in, 1 out]
                n2150 = call "Write flatted cluster.vi"("error in (no error)"=w4255, "flatted cluster"=w4254, "Interface in"=w4263) -> ("error out"=w4265:errorcluster, "Interface out"=w4264:refnum<class "Interface.lvclass">)  [unwired: 7 in]
                n2151 = call-dynamic "Write Interface.vi"("error in (no error)"=w4265, "Interface.lvclass"=w4264, "Channel in"=w4250) -> ("error out"=w4271:errorcluster, "Channel out"=w4272:refnum<class "Channel.lvclass">)  [unwired: 7 in]
                n2152 = call "Write section_name.vi"("error in (no error)"=w4271, "section_name"="CCD_ACS3", "Channel in"=w4272) -> ("error out"=w4269:errorcluster, "Channel out"=w4275:refnum<class "Channel.lvclass">)  [unwired: 7 in]
                n2153 = call-dynamic "save config.vi"("error in (no error)"=w4269, "file config"="lastsaved.cfg", "Channel in"=w4275) -> ("error out"=w4270:errorcluster, "Channel out"=w4276:refnum<class "Channel.lvclass">)  [unwired: 7 in]
                n2154 = call-dynamic "Read State Machine.vi"("error in (no error)"=w4270, "Device in"=w4276) -> ("error out"=w4266:errorcluster, "State Machine.lvclass"=w4278:refnum<class "State Machine.lvclass">, "Device out"=w4277:refnum<class "Channel.lvclass">)  [unwired: 7 in]
                n2155 = call-dynamic "Write State.vi"("error in (no error)"=w4266, "State"=60, "State Machine in"=w4278) -> ("error out"=w4267:errorcluster, "State Machine out"=w4279:refnum<class "State Machine.lvclass">)  [unwired: 7 in]
                n2156 = call-dynamic "Write State Machine.vi"("error in (no error)"=w4267, "State Machine.lvclass"=w4279, "Device in"=w4277) -> ("error out"=w4281:errorcluster, "Device out"=w4280:refnum<class "Channel.lvclass">)  [unwired: 7 in]
                n2157 = call-dynamic "Write Channel.vi"("error in (no error)"=w4281, "Channel.lvclass"=w4280, "Acquisition in"=w4251) -> ("error out"=w4246:errorcluster, "Acquisition out"=w4247:refnum<class "Acquisition.lvclass">)  [unwired: 7 in]
              }
            }
            n2158 = case shown="True" w4186 {
              tunnel: w4188 -> [w4205 w4210]
              tunnel: w4187 -> [w4204 w4209]
              tunnel: [w4205 w4208] -> w4159
              tunnel: [w4204 w4207] -> w4158
              tunnel: w4156 -> [_ w4206]
              frame False {
              }
              frame True {
                # "nome do arquivo .cfg"
                # "seção no arquivo .cfg"
                n2159 = call-dynamic "Read Channel.vi"("error in (no error)"=w4209, "Acquisition in"=w4210) -> ("error out"=w4239:errorcluster, "Channel.lvclass"=w4240:refnum<class "Channel.lvclass">, "Acquisition out"=w4241:refnum<class "Acquisition.lvclass">)  [unwired: 7 in]
                n2160 = call-dynamic "Read Interface.vi"("error in (no error)"=w4239, "Channel in"=w4240) -> ("error out"=w4232:errorcluster, "Interface.lvclass"=w4231:refnum<class "Interface.lvclass">, "Channel out"=w4242:refnum<class "Channel.lvclass">)  [unwired: 7 in]
                n2161 = call-dynamic "Get CCD_Config.vi"("error in (no error)"=w4232, "Interface in"=w4231) -> ("error out"=w4234:errorcluster, "output cluster"=w4235:T31, "Interface out"=w4230:refnum<class "Interface.lvclass">)  [unwired: 7 in]
                n2162 = Bundle By Name(cluster=w4235, "TRIGGER_MODE"=w4206) -> (w4233:T31)
                n2163 = call-dynamic "Set CCD_Config.vi"("error in (no error)"=w4234, "input cluster"=w4233, "Interface in"=w4230) -> ("error out"=w4236:errorcluster, "Interface out"=w4229:refnum<class "Interface.lvclass">)  [unwired: 7 in]
                n2164 = Flatten To String(anything=w4233, error in (no error)=w4236) -> (data string=w4238:string, error out=w4237:errorcluster)  [unwired: 2 in, 1 out]
                n2165 = call "Write flatted cluster.vi"("error in (no error)"=w4237, "flatted cluster"=w4238, "Interface in"=w4229) -> ("error out"=w4227:errorcluster, "Interface out"=w4228:refnum<class "Interface.lvclass">)  [unwired: 7 in]
                n2166 = call-dynamic "Write Interface.vi"("error in (no error)"=w4227, "Interface.lvclass"=w4228, "Channel in"=w4242) -> ("error out"=w4221:errorcluster, "Channel out"=w4220:refnum<class "Channel.lvclass">)  [unwired: 7 in]
                n2167 = call "Write section_name.vi"("error in (no error)"=w4221, "section_name"="CCD_ACS4", "Channel in"=w4220) -> ("error out"=w4223:errorcluster, "Channel out"=w4217:refnum<class "Channel.lvclass">)  [unwired: 7 in]
                n2168 = call-dynamic "save config.vi"("error in (no error)"=w4223, "file config"="lastsaved.cfg", "Channel in"=w4217) -> ("error out"=w4222:errorcluster, "Channel out"=w4216:refnum<class "Channel.lvclass">)  [unwired: 7 in]
                n2169 = call-dynamic "Read State Machine.vi"("error in (no error)"=w4222, "Device in"=w4216) -> ("error out"=w4226:errorcluster, "State Machine.lvclass"=w4214:refnum<class "State Machine.lvclass">, "Device out"=w4215:refnum<class "Channel.lvclass">)  [unwired: 7 in]
                n2170 = call-dynamic "Write State.vi"("error in (no error)"=w4226, "State"=60, "State Machine in"=w4214) -> ("error out"=w4225:errorcluster, "State Machine out"=w4213:refnum<class "State Machine.lvclass">)  [unwired: 7 in]
                n2171 = call-dynamic "Write State Machine.vi"("error in (no error)"=w4225, "State Machine.lvclass"=w4213, "Device in"=w4215) -> ("error out"=w4211:errorcluster, "Device out"=w4212:refnum<class "Channel.lvclass">)  [unwired: 7 in]
                n2172 = call-dynamic "Write Channel.vi"("error in (no error)"=w4211, "Channel.lvclass"=w4212, "Acquisition in"=w4241) -> ("error out"=w4207:errorcluster, "Acquisition out"=w4208:refnum<class "Acquisition.lvclass">)  [unwired: 7 in]
              }
            }
            n2173 = case shown="True" w4192 {
              tunnel: w4194 -> [w4283 w4288]
              tunnel: w4193 -> [w4282 w4287]
              tunnel: [w4283 w4286] -> w4163
              tunnel: [w4282 w4285] -> w4162
              tunnel: w4156 -> [_ w4284]
              frame False {
              }
              frame True {
                # "nome do arquivo .cfg"
                # "seção no arquivo .cfg"
                n2174 = call-dynamic "Read Channel.vi"("error in (no error)"=w4287, "Acquisition in"=w4288) -> ("error out"=w4292:errorcluster, "Channel.lvclass"=w4291:refnum<class "Channel.lvclass">, "Acquisition out"=w4290:refnum<class "Acquisition.lvclass">)  [unwired: 7 in]
                n2175 = call-dynamic "Read Interface.vi"("error in (no error)"=w4292, "Channel in"=w4291) -> ("error out"=w4299:errorcluster, "Interface.lvclass"=w4300:refnum<class "Interface.lvclass">, "Channel out"=w4289:refnum<class "Channel.lvclass">)  [unwired: 7 in]
                n2176 = call-dynamic "Get CCD_Config.vi"("error in (no error)"=w4299, "Interface in"=w4300) -> ("error out"=w4297:errorcluster, "output cluster"=w4296:T31, "Interface out"=w4301:refnum<class "Interface.lvclass">)  [unwired: 7 in]
                n2177 = Bundle By Name(cluster=w4296, "TRIGGER_MODE"=w4284) -> (w4298:T31)
                n2178 = call-dynamic "Set CCD_Config.vi"("error in (no error)"=w4297, "input cluster"=w4298, "Interface in"=w4301) -> ("error out"=w4295:errorcluster, "Interface out"=w4302:refnum<class "Interface.lvclass">)  [unwired: 7 in]
                n2179 = Flatten To String(anything=w4298, error in (no error)=w4295) -> (data string=w4293:string, error out=w4294:errorcluster)  [unwired: 2 in, 1 out]
                n2180 = call "Write flatted cluster.vi"("error in (no error)"=w4294, "flatted cluster"=w4293, "Interface in"=w4302) -> ("error out"=w4304:errorcluster, "Interface out"=w4303:refnum<class "Interface.lvclass">)  [unwired: 7 in]
                n2181 = call-dynamic "Write Interface.vi"("error in (no error)"=w4304, "Interface.lvclass"=w4303, "Channel in"=w4289) -> ("error out"=w4310:errorcluster, "Channel out"=w4311:refnum<class "Channel.lvclass">)  [unwired: 7 in]
                n2182 = call "Write section_name.vi"("error in (no error)"=w4310, "section_name"="CCD_ACS2", "Channel in"=w4311) -> ("error out"=w4308:errorcluster, "Channel out"=w4314:refnum<class "Channel.lvclass">)  [unwired: 7 in]
                n2183 = call-dynamic "save config.vi"("error in (no error)"=w4308, "file config"="lastsaved.cfg", "Channel in"=w4314) -> ("error out"=w4309:errorcluster, "Channel out"=w4315:refnum<class "Channel.lvclass">)  [unwired: 7 in]
                n2184 = call-dynamic "Read State Machine.vi"("error in (no error)"=w4309, "Device in"=w4315) -> ("error out"=w4305:errorcluster, "State Machine.lvclass"=w4317:refnum<class "State Machine.lvclass">, "Device out"=w4316:refnum<class "Channel.lvclass">)  [unwired: 7 in]
                n2185 = call-dynamic "Write State.vi"("error in (no error)"=w4305, "State"=60, "State Machine in"=w4317) -> ("error out"=w4306:errorcluster, "State Machine out"=w4318:refnum<class "State Machine.lvclass">)  [unwired: 7 in]
                n2186 = call-dynamic "Write State Machine.vi"("error in (no error)"=w4306, "State Machine.lvclass"=w4318, "Device in"=w4316) -> ("error out"=w4320:errorcluster, "Device out"=w4319:refnum<class "Channel.lvclass">)  [unwired: 7 in]
                n2187 = call-dynamic "Write Channel.vi"("error in (no error)"=w4320, "Channel.lvclass"=w4319, "Acquisition in"=w4290) -> ("error out"=w4285:errorcluster, "Acquisition out"=w4286:refnum<class "Acquisition.lvclass">)  [unwired: 7 in]
              }
            }
            n2188 = case shown="True" w4195 {
              tunnel: [w4321 w4355] -> w4164
              tunnel: [w4322 w4354] -> w4165
              tunnel: w4197 -> [w4322 w4325]
              tunnel: w4196 -> [w4321 w4324]
              tunnel: w4156 -> [_ w4323]
              frame False {
              }
              frame True {
                # "nome do arquivo .cfg"
                # "seção no arquivo .cfg"
                n2189 = call-dynamic "Read Channel.vi"("error in (no error)"=w4324, "Acquisition in"=w4325) -> ("error out"=w4356:errorcluster, "Channel.lvclass"=w4357:refnum<class "Channel.lvclass">, "Acquisition out"=w4358:refnum<class "Acquisition.lvclass">)  [unwired: 7 in]
                n2190 = call-dynamic "Read Interface.vi"("error in (no error)"=w4356, "Channel in"=w4357) -> ("error out"=w4347:errorcluster, "Interface.lvclass"=w4346:refnum<class "Interface.lvclass">, "Channel out"=w4359:refnum<class "Channel.lvclass">)  [unwired: 7 in]
                n2191 = call-dynamic "Get CCD_Config.vi"("error in (no error)"=w4347, "Interface in"=w4346) -> ("error out"=w4349:errorcluster, "output cluster"=w4350:T31, "Interface out"=w4345:refnum<class "Interface.lvclass">)  [unwired: 7 in]
                n2192 = Bundle By Name(cluster=w4350, "TRIGGER_MODE"=w4323) -> (w4348:T31)
                n2193 = call-dynamic "Set CCD_Config.vi"("error in (no error)"=w4349, "input cluster"=w4348, "Interface in"=w4345) -> ("error out"=w4351:errorcluster, "Interface out"=w4344:refnum<class "Interface.lvclass">)  [unwired: 7 in]
